vi "turret_periodic.vi"(10 "Enable Turret":bool) -> ()   [LabVIEW 2020]
uses:
  <vilib>/Rock Robotics/WPI/ThirdParty/Phoenix-LabVIEW/Motor Controller/Controls/CTRE_Phoenix_MotorControl_ControlMode.ctl
  <vilib>/Rock Robotics/WPI/ThirdParty/Phoenix-LabVIEW/Motor Controller/Get/CTRE_Phoenix_MotorController_GetSelectedSensorData.vi
  <vilib>/Rock Robotics/Network Tables/NT Write Number.vi
  <vilib>/Rock Robotics/Network Tables/NT Read Number.vi
  <vilib>/Rock Robotics/WPI/ThirdParty/Phoenix-LabVIEW/Motor Controller/Get/CTRE_Phoenix_MotorController_GetVoltage.vi
  TitanLib/Lib/TitanLib.lvlib
panel:
  out "Invalid Target":bool
  out "ty":dbl
  out "Turret out of range":bool
  out "Turret Theta (Deg)":dbl
  out "Target Distance (in)":dbl
  in  "Turret Override":bool
  in  "Override Setpoint":dbl
  out "Percent Output":dbl(graph)
  out "Setpoint (Deg)":dbl format="%.2f"
  in  "Turret Constants":T1={"Set Constants"=FALSE, "P"=0.05, "I"=0.0, "D"=0.0, "F"=0.0, "I Zone"=0.0, "Cruise Velocity"=500000, "Acceleration"=500000, "Percent Deadband"=0.0}
  out "tx":dbl
  out "Current Position (Deg)":dbl format="%.2f"
  in  "Zero Turret Encoder":bool
  in  "Min Rotation (deg)":dbl=-45.0
  in  "Max Rotation (deg)":dbl=20.0
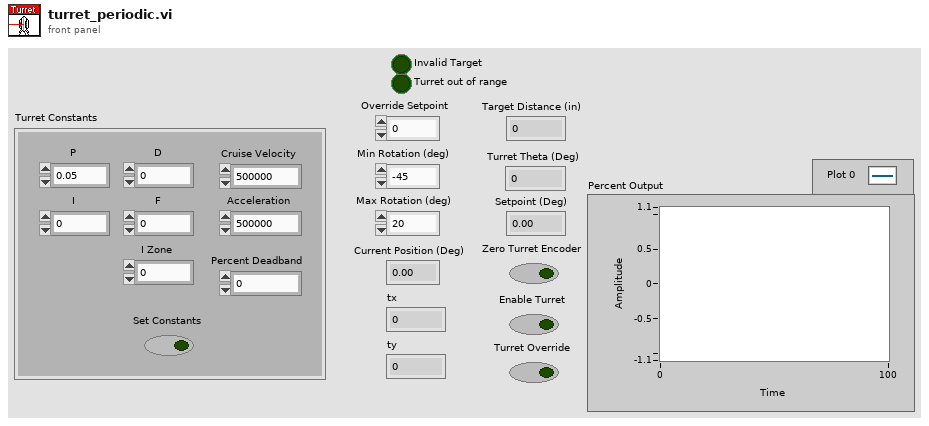
[diagram p1: front panel]
types:
  T1 = cluster{"Set Constants":bool, "P":dbl, "I":dbl, "D":dbl, "F":dbl, "I Zone":dbl, "Cruise Velocity":i32, "Acceleration":i32, "Percent Deadband":dbl}
  T2 = typedef "WPI_MotorControlDeviceRef.ctl" = cluster{"DeviceStatus":errorcluster, "Type":T3, "PWM":cluster{"PWM Channel":T4, "DeadBand":T5}, "CAN":cluster{"Device Number":u8, "SetOutput VI Ref":variant, "GetOutput VI Ref":variant, "Enable VI Ref":variant, "Disable VI Ref":variant, "Data":variant}, "Invert":bool, "DIO PWM":cluster{"PWM \"Enable\" Channel":T4, "DIOChannel":T6, "PWM Rate":dbl}}
  T3 = typedef "WPI_MotorControlType.ctl" = enum16{"PWM", "CAN", "DIO PWM"}
  T4 = typedef "FPGA_DIOPWMChannel.ctl" = enum8{"PWM 0", "PWM 1", "PWM 2", "PWM 3", "PWM 4", "PWM 5", "PWM 6", "PWM 7", "PWM 8", "PWM 9", "PWM MXP 0", "PWM MXP 1", "PWM MXP 2", "PWM MXP 3", "PWM MXP 4", "PWM MXP 5", "PWM MXP 6", "PWM MXP 7", "PWM MXP 8", "PWM MXP 9", "Invalid"}
  T5 = typedef "WPI_PWMDeadband.ctl" = cluster{"Name":string, "maxPositivePwm":i32, "minPositivePwm":i32, "centerPwm":i32, "maxNegativePwm":i32, "minNegativePwm":i32, "angularRange":u16}
  T6 = typedef "FPGA_DIOChannel.ctl" = enum8{"DIO 0", "DIO 1", "DIO 2", "DIO 3", "DIO 4", "DIO 5", "DIO 6", "DIO 7", "DIO 8", "DIO 9", "DIO MXP 0", "DIO MXP 1", "DIO MXP 2", "DIO MXP 3", "DIO MXP 4", "DIO MXP 5", "DIO MXP 6", "DIO MXP 7", "DIO MXP 8", "DIO MXP 9", "DIO MXP 10", "DIO MXP 11", "DIO MXP 12", "DIO MXP 13", "DIO MXP 14", "DIO MXP 15", "SPI Port CS1", "SPI Port CS2", "SPI Port CS3", "SPI Port MISO", "SPI Port MOSI", "Invalid"}
  T7 = typedef "CTRE_Phoenix_MotorControl_ControlMode.ctl" = u16
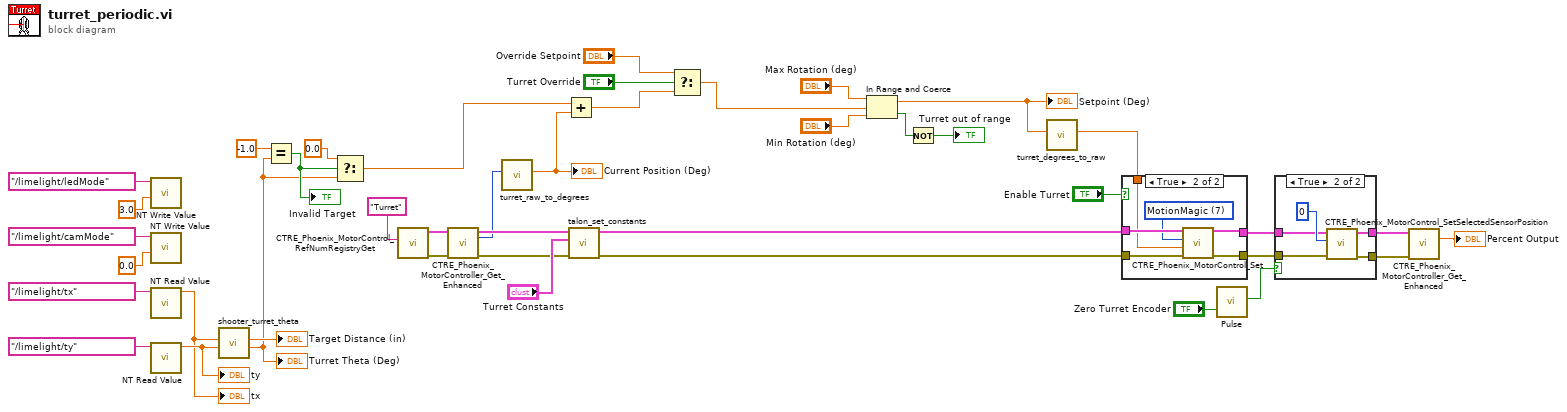
[diagram p0: block diagram]
diagram:
  n1 = call-poly <vilib>:"NT Write Value.vi"("Numeric"=3.0, "Name"="/limelight/ledMode") -> ()  [unwired: 9 in, 1 out]
  n2 = call-poly <vilib>:"NT Write Value.vi"("Numeric"=0.0, "Name"="/limelight/camMode") -> ()  [unwired: 9 in, 1 out]
  n3 = call-poly <vilib>:"NT Read Value.vi"("Name"="/limelight/tx") -> ("Numeric"=w9:dbl)  [unwired: 9 in, 1 out]
  "tx" <- w9
  n4 = call-poly <vilib>:"NT Read Value.vi"("Name"="/limelight/ty") -> ("Numeric"=w22:dbl)  [unwired: 9 in, 1 out]
  "ty" <- w22
  n5 = call "shooter_turret_theta.vi"("Target y (Deg)"=w22, "Target x (deg)"=w9) -> ("Theta"=w4:dbl, "Target Distance (in)"=→"Target Distance (in)":dbl)  [unwired: 8 in]
  "Turret Theta (Deg)" <- w4
  n6 = Equal?(x=-1.0 ("y"), y=w4) -> (x = y?=w6:bool)
  "Invalid Target" <- w6
  n7 = Select(t=0.0, s=w6, f=w4) -> (s? t:f=w3:dbl)
  n8 = call <vilib>:"CTRE_Phoenix_MotorControl_RefNumRegistryGet.vi"("refnum name"="Turret") -> ("error out"=w32:errorcluster, "PhoenixMotorControlDevRef"=w33:T2)  [unwired: 9 in]
  n9 = call-poly <vilib>:"CTRE_Phoenix_MotorController_Get_Enhanced.vi"("PhoenixMotorControlDevRef"=w33, "error in"=w32) -> ("PhoenixMotorControlDevRef"=w20:T2, "Position (Raw Sensor Units)"=w15:i32, "error out"=w19:errorcluster)  [unwired: 10 in, 1 out]
  n10 = call "turret_raw_to_degrees.vi"("Raw Encoder Units In"=w15) -> ("Degrees Out"=w12:dbl)  [unwired: 10 in]
  "Current Position (Deg)" <- w12
  n11 = Add(x=w3, y=w12) -> (x+y=w2:dbl)
  n12 = call "talon_set_constants.vi"("error in"=w19, "Constants"="Turret Constants", "PhoenixMotorControlDevRef"=w20) -> ("error out"=w30:errorcluster, "PhoenixMotorControlDevRef"=w31:T2)  [unwired: 7 in]
  n13 = Select(t="Override Setpoint", s="Turret Override", f=w2) -> (s? t:f=w1:dbl)
  n14 = In Range and Coerce(upper limit="Max Rotation (deg)", x=w1, lower limit="Min Rotation (deg)") -> (coerced(x)=w8:dbl, In Range?=w11:bool)
  "Setpoint (Deg)" <- w8
  n15 = Not(x=w11) -> (.not. x?=→"Turret out of range":bool)
  n16 = call "turret_degrees_to_raw.vi"("Degrees In"=w8) -> ("Raw Encoder Units Out"=w7:dbl)  [unwired: 10 in]
  n17 = case shown="True" "Enable Turret" {
    tunnel: w31 -> [w44 w50]
    tunnel: w30 -> [w43 w49]
    tunnel: [w44 w48] -> w41
    tunnel: [w43 w47] -> w40
    tunnel: w7 -> [_ w45]
    frame False {
    }
    frame True {
      w46 = T7 7 items=["PercentOutput"=0, "Position"=1, "Velocity"=2, "Current"=3, "Follower"=5, "MotionProfile"=6, "MotionMagic"=7, "MotionProfileArc"=10, "Disabled"=15] ("Control Mode")
      n18 = call <vilib>:"CTRE_Phoenix_MotorControl_Set.vi"("error in (no error)"=w49, "Output"=w45, "Control Mode"=w46, "PhoenixMotorControlDevRef"=w50) -> ("error out"=w47:errorcluster, "PhoenixMotorControlDevRef"=w48:T2)  [unwired: 6 in]
    }
  }
  n19 = call "Pulse.vi"("Input"="Zero Turret Encoder") -> ("Output"=w39:bool)  [unwired: 10 in]
  n20 = case shown="True" w39 {
    tunnel: w41 -> [w52 w56]
    tunnel: w40 -> [w51 w55]
    tunnel: [w52 w54] -> w18
    tunnel: [w51 w53] -> w17
    frame False {
    }
    frame True {
      n21 = call <vilib>:"CTRE_Phoenix_MotorControl_SetSelectedSensorPosition.vi"("error in (no error)"=w55, "New Sensor Position"=0, "PhoenixMotorControlDevRef"=w56) -> ("error out"=w53:errorcluster, "PhoenixMotorControlDevRef"=w54:T2)  [unwired: 7 in]
    }
  }
  n22 = call-poly <vilib>:"CTRE_Phoenix_MotorController_Get_Enhanced.vi"("PhoenixMotorControlDevRef"=w18, "error in"=w17) -> ("Percent Output"=→"Percent Output":dbl)  [unwired: 9 in, 4 out]
